vi "fahrenheitToCentigrade.vi"(9 "Convert?":bool, 10 "Schedule Before":T2(array[cluster])) -> (2 "Schedule After":T1(array[cluster]))   [LabVIEW 2018]
panel:
  # "True: Output Rate is Converted From Fahrenheit to Celcius\nFalse: Output Rate Remains Unchanged"
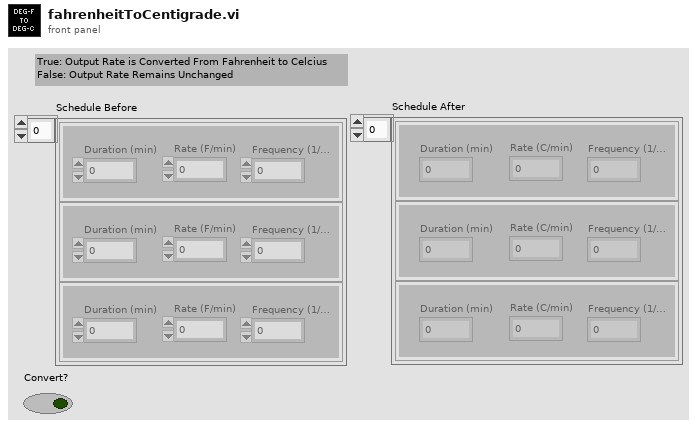
[diagram p1: front panel]
types:
  T1 = cluster{"Duration (min)":dbl, "Rate (C/min) ":dbl, "Frequency (1/min)":dbl}[]
  T2 = cluster{"Duration (min)":dbl, "Rate (F/min) ":dbl, "Frequency (1/min)":dbl}[]
  T3 = cluster{"Duration (min)":dbl, dbl, "Frequency (1/min)":dbl}
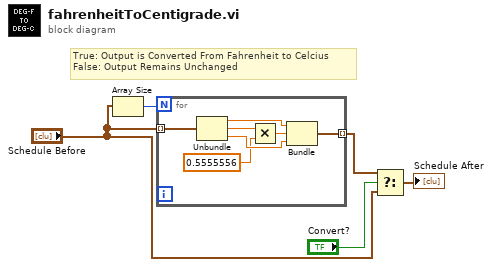
[diagram p0: block diagram]
diagram:
  # "True: Output is Converted From Fahrenheit to Celcius\nFalse: Output Remains Unchanged"
  n1 = Array Size(array="Schedule Before") -> (size(s)=w5:i32)
  n2 = for {
    N: w5 -> [_]
    tunnel: "Schedule Before" -> [w12] mode=indexing
    tunnel: [w9] -> w2 mode=indexing
    n3 = Unbundle(w12) -> ("Duration (min)"=w11:dbl, "Rate (F/min)"=w7:dbl, "Frequency (1/min)"=w10:dbl)
    n4 = Multiply(x=w7, y=0.5555556) -> (x*y=w6:dbl)
    n5 = Bundle("Duration (min)"=w11, w6, "Frequency (1/min)"=w10) -> (w9:T3)  [unwired: 1 in]
  }
  n6 = Select(t=w2, s="Convert?", f="Schedule Before") -> (s? t:f=→"Schedule After":T2)
